vi "rtlsdr_read_array_of_IQ.vi"(7 "ref in":refnum<k5>, 8 "error in (no error)":errorcluster, 9 "buffer size":i32=1024, 10 "index":u32, 11 "array in":cluster{"I sample":u8, "Q sample":u8}[](array[cluster])) -> (0 "error out":errorcluster, 2 "next index":u32, 3 "array out":cluster{"I sample":u8, "Q sample":u8}[](array[cluster]), 5 "ref out":refnum<k5>)   [LabVIEW 2011]
doc: "Az I/Q adatokat olvassa le az RTL-SDR eszközrõl. A kimenet Cluster-ek tömbje."
panel:
  # "Outputs:"
  # "Inputs:"
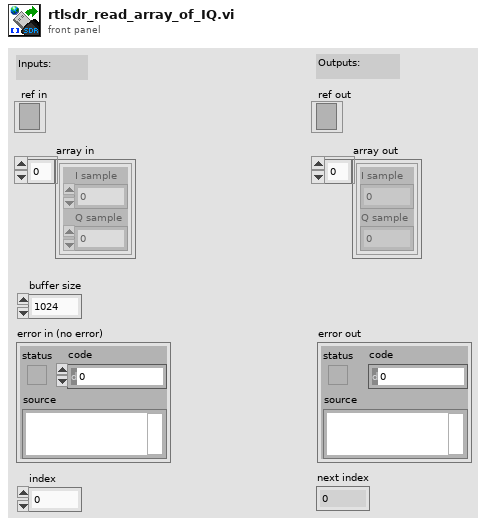
[diagram p1: front panel]
types:
  T1 = enum16{"Standard", "Buffered", "CRLF", "Immediate"}
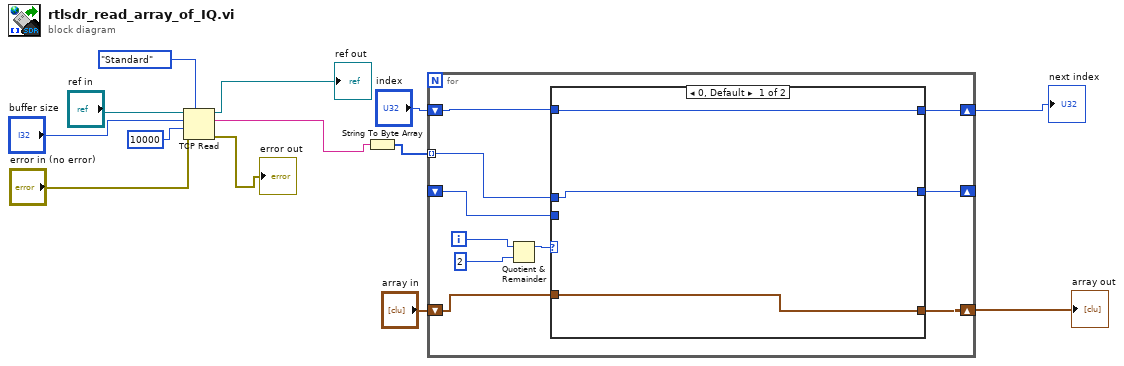
[diagram p0: block diagram]
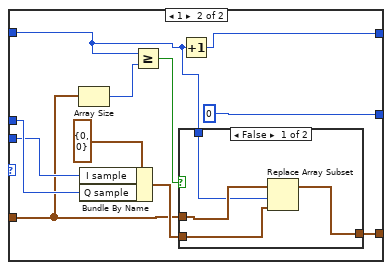
[diagram p2: hidden frame]
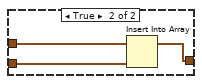
[diagram p3: hidden frame]
diagram:
  n1 = TCP Read(connection ID="ref in", bytes to read="buffer size", error in (no error)="error in (no error)", 7:T1."Standard" ("mode (standard)"), 9:10000 ("timeout ms (25000)")) -> (connection ID out=→"ref out":refnum<k5>, data out=w8:string, error out=→"error out":errorcluster)
  n2 = String To Byte Array(string=w8) -> (unsigned byte array=w7:u8[])
  n3 = for {
    tunnel: w7 -> [w20] mode=indexing
    shift-right: [w19] -> _
    shift-left: _ -> [w18]
    shift-right: [w16] -> w5
    shift-left: "array in" -> [w17]
    shift-right: [w14] -> w1
    shift-left: "index" -> [w15]
    i -> [w23]
    n4 = Quotient & Remainder(x=w23, y=2) -> (x-y*floor(x/y)=w21:i32)  [unwired: 1 out]
    n5 = case shown="0, Default" w21 {
      tunnel: w20 -> [w26 w36]
      tunnel: [w26 u8 0] -> w19
      tunnel: w18 -> [_ w35]
      tunnel: w17 -> [w25 w31]
      tunnel: [w25 w32] -> w16
      tunnel: w15 -> [w24 w27]
      tunnel: [w24 w28] -> w14
      frame 0, Default {
      }
      frame 1 {
        n6 = Array Size(array=w31) -> (size(s)=w29:i32)
        n7 = Bundle By Name(cluster=cluster{"I sample":u8, "Q sample":u8} {"I sample"=0, "Q sample"=0} ("I/Q sample cluster"), "I sample"=w35, "Q sample"=w36) -> (w33:cluster{"I sample":u8, "Q sample":u8})
        n8 = Greater Or Equal?(x=w27, y=w29) -> (x >= y?=w30:bool)
        n9 = case shown="False" w30 {
          tunnel: w33 -> [w39 w44]
          tunnel: w31 -> [w41 w43]
          tunnel: [w38 w42] -> w32
          tunnel: w27 -> [w40 _]
          frame False {
            n10 = Replace Array Subset(array=w41, new element=w39, index=w40) -> (w38:cluster{"I sample":u8, "Q sample":u8}[])
          }
          frame True {
            n11 = Insert Into Array(array=w43, new element=w44) -> (w42:cluster{"I sample":u8, "Q sample":u8}[])  [unwired: 1 in]
          }
        }
        n12 = Increment(x=w27) -> (x+1=w28:u32)
      }
    }
  }
  "array out" <- w5
  "next index" <- w1
